vi "Power on DVDD.vi"   [LabVIEW 2010]
uses:
  <instrlib>/Keithley 2400/Keithley 24XX.lvlib
types:
  T1 = typedef "niSE SessionRefnum.ctl" = refnum<k1>
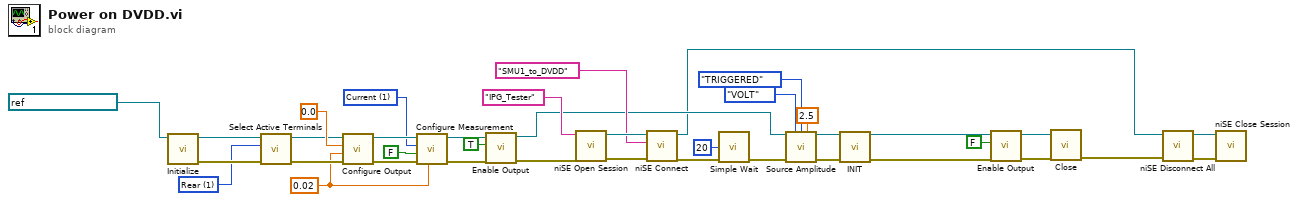
[diagram p0: block diagram]
diagram:
  w29 = u16 1 items=["Volts", "Current", "Resistance"] ("Function (0: Volts)")
  w32 = u16 1 items=["Front", "Rear"] ("Active Terminals (0: Front)")
  w24 = 0.02 ("Compliance  Level (0.1)")
  n1 = call <instrlib>:"Initialize.vi"("VISA resource name"=refnum<visa-resource-name> "GPIB0::9::INSTR") -> ("error out"=w34:errorcluster, "VISA resource name out"=w36:refnum<visa-resource-name>)  [unwired: 9 in]
  n2 = call <instrlib>:"Select Active Terminals.vi"("error in (no error)"=w34, "Active Terminals (0: Front)"=w32, "VISA resource name"=w36) -> ("error out"=w33:errorcluster, "VISA resource name out"=w35:refnum<visa-resource-name>)  [unwired: 7 in]
  n3 = call <instrlib>:"Configure Output.vi"("error in (no error)"=w33, "Compliance  Level (0.1)"=w24, "Output Level (0)"=0.0, "VISA resource name"=w35) -> ("error out"=w30:errorcluster, "VISA resource name out"=w31:refnum<visa-resource-name>)  [unwired: 6 in]
  n4 = call <instrlib>:"Configure Measurement.vi"("Manual Range (1.0)"=w24, "error in (no error)"=w30, "Enable Auto Range (T:Enable)"=FALSE, "Function (0: Volts)"=w29, "VISA resource name"=w31) -> ("error out"=w26:errorcluster, "VISA resource name out"=w27:refnum<visa-resource-name>)  [unwired: 5 in]
  n5 = call <instrlib>:"Enable Output.vi"("error in (no error)"=w26, "Enable Output (T: Enable)"=TRUE, "VISA resource name"=w27) -> ("error out"=w15:errorcluster, "VISA resource name out"=w12:refnum<visa-resource-name>)  [unwired: 7 in]
  n6 = call <vilib>:"niSE Open Session.vi"("error in (no error)"=w15, "Virtual Device Name (SwitchConfiguration1)"="IPG_Tester") -> ("error out"=w14:errorcluster, "NISE Session (out)"=w23:T1)  [unwired: 4 in]
  n7 = call <vilib>:"niSE Connect.vi"("error in (no error)"=w14, "Connection Specification (\"\")"="SMU1_to_DVDD" ("Connection Specification (\"\")"), "NISE Session (in)"=w23) -> ("error out"=w13:errorcluster, "NISE Session (out)"=w4:T1)  [unwired: 7 in]
  n8 = call "Simple Wait.vi"("mS"=u32 20, "error in"=w13) -> ("error out"=w16:errorcluster)  [unwired: 12 in, 1 out]
  n9 = call "Source Amplitude.vi"("VISA resource name"=w12, "Source Function"=enum16{"CURR", "VOLT"}."VOLT", "Mode"=enum16{"IMM", "TRIGGERED"}."TRIGGERED", "Source Level"=2.5, "error in (no error)"=w16) -> ("VISA resource name out"=w19:refnum<visa-resource-name>, "error out"=w18:errorcluster)  [unwired: 9 in]
  n10 = call "INIT.vi"("VISA resource name"=w19, "error in (no error)"=w18) -> ("VISA resource name out"=w3:refnum<visa-resource-name>, "error out"=w2:errorcluster)  [unwired: 12 in]
  n11 = call <instrlib>:"Enable Output.vi"("error in (no error)"=w2, "Enable Output (T: Enable)"=FALSE, "VISA resource name"=w3) -> ("error out"=w6:errorcluster, "VISA resource name out"=w5:refnum<visa-resource-name>)  [unwired: 7 in]
  n12 = call <instrlib>:"Close.vi"("error in (no error)"=w6, "VISA resource name"=w5) -> ("error out"=w1:errorcluster)  [unwired: 9 in]
  n13 = call <vilib>:"niSE Disconnect All.vi"("error in (no error)"=w1, "NISE Session (in)"=w4) -> ("error out"=w9:errorcluster, "NISE Session (out)"=w8:T1)  [unwired: 4 in]
  n14 = call <vilib>:"niSE Close Session.vi"("error in (no error)"=w9, "NISE Session (in)"=w8) -> ()  [unwired: 5 in, 1 out]
